vi "Info.vi"(8 "error in":errorcluster, 11 "VISA resource name":refnum<visa-resource-name>) -> (0 "error out\n(to Instr. Write/Read.vi)":errorcluster, 3 "VISA resource name out":refnum<visa-resource-name>)   [LabVIEW 2016, in "Agilent 415X Series.lvlib"]
doc: "This VI describes how to perform parameter range error checking if the user so desires to implement it."
uses:
  Agilent 415X Series.lvlib
panel:
  in  "x control":dbl format="%.2f"
  in  "revision history":string
  in  "by":string="Instrument Driver Development Team, National Instruments"
  in  "options":string="none (no HP16440A, HP16441A, HP16442A, or HP41501A"
  in  "comminication":u16(ring) items=["GPIB", "VXIbus", "Serial"]
  in  "firmware revision (*IDN?)":string="01.00:01.00:01.00"
  in  "manual revision or p/n":string="PN 04155-90120"
  in  "?":string="HP4155A Semiconductor Parameter Analyzer"
  # "instrument"
  # "instrument driver"
  # "more ..\n(see diagram)"
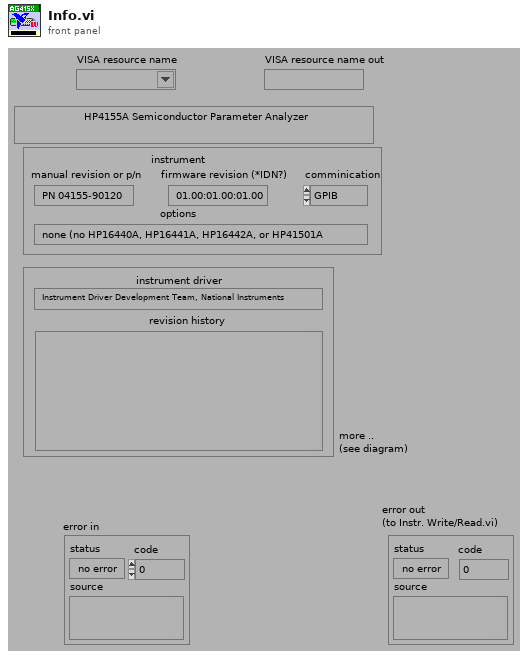
[diagram p1: front panel]
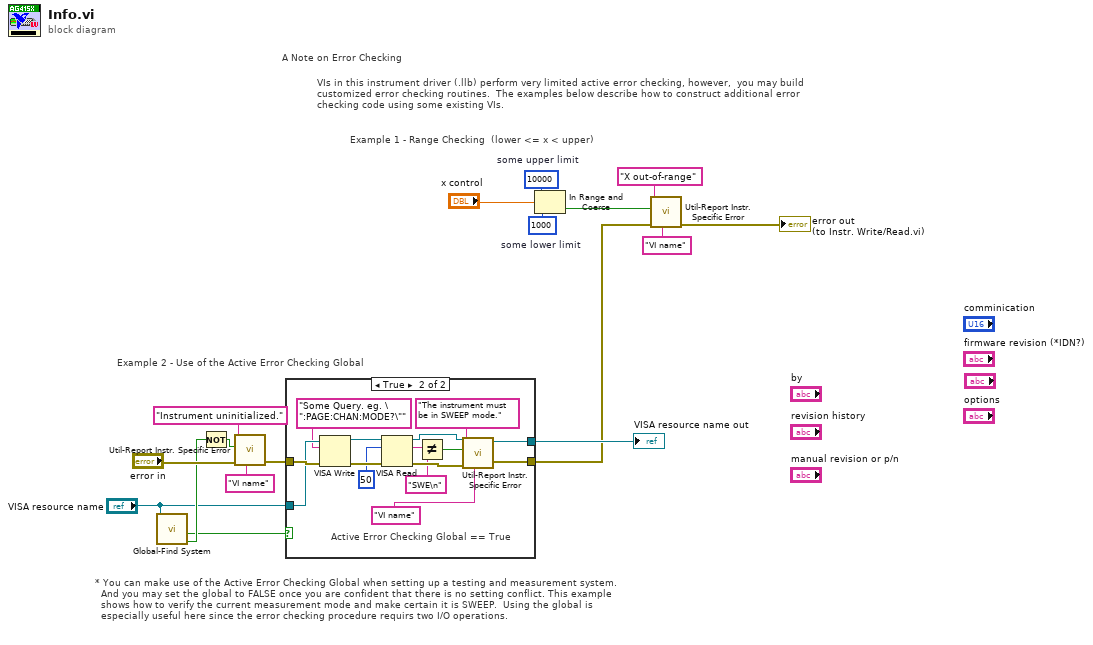
[diagram p0: block diagram]
diagram:
  w13 = 1000  # some lower limit
  w12 = 10000  # some upper limit
  # "A Note on Error Checking"
  # "* You can make use of the Active Error Checking Global when setting up a testing and measurement system.\n  And you may set the global to FALSE once you are confident that there is no setting conflict. This example\n  shows how to verify the current measurement mode and make certain it is SWEEP.  Using the global is  \n  especially useful here since the error checking procedure requirs two I/O operations."
  # "Example 2 - Use of the Active Error Checking Global"
  # "Example 1 - Range Checking  (lower <= x < upper)"
  # "VIs in this instrument driver (.llb) perform very limited active error checking, however,  you may build\ncustomized error checking routines.  The examples below describe how to construct additional error\nchecking code using some existing VIs."
  n1 = call "Global-Find System.vi"("VISA session"="VISA resource name") -> ("found"=w9:bool, "active error checking"=w6:bool)  [unwired: 3 in, 6 out]
  n2 = Not(x=w9) -> (.not. x?=w10:bool)
  n3 = call "Util-Report Instr. Specific Error.vi"("source"="VI name", "error in (no error)"="error in", "error message"="Instrument uninitialized.", "new error"=w10) -> ("error out"=w5:errorcluster)  [unwired: 6 in, 1 out]
  n4 = case shown="True" w6 {
    tunnel: w5 -> [w19 w34]
    tunnel: [w19 w25] -> w2
    tunnel: "VISA resource name" -> [w18 w32]
    tunnel: [w18 w20] -> w3
    frame False {
      # "Active Error Checking Global == False"
    }
    frame True {
      # "Active Error Checking Global == True"
      n5 = VISA Write(VISA resource name=w32, write buffer="Some Query. eg. \":PAGE:CHAN:MODE?\"", error in (no error)=w34) -> (VISA resource name out=w31:refnum<visa-resource-name>, error out=w33:errorcluster)  [unwired: 1 out]
      n6 = VISA Read(VISA resource name=w31, byte count=50, error in (no error)=w33) -> (VISA resource name out=w21:refnum<visa-resource-name>, read buffer=w28:string, error out=w26:errorcluster)  [unwired: 1 out]
      n7 = Not Equal?(x=w28, y="SWE\n") -> (x != y?=w27:bool)
      n8 = call "Util-Report Instr. Specific Error.vi"("source"="VI name", "error in (no error)"=w26, "error message"="The instrument must be in SWEEP mode.", "new error"=w27, "VISA resource name"=w21) -> ("error out"=w25:errorcluster, "VISA resource name out"=w20:refnum<visa-resource-name>)  [unwired: 5 in]
    }
  }
  "VISA resource name out" <- w3
  n9 = In Range and Coerce(upper limit=w12, x="x control", lower limit=w13) -> (In Range?=w17:bool)  [unwired: 1 out]
  n10 = call "Util-Report Instr. Specific Error.vi"("source"="VI name", "error in (no error)"=w2, "error message"="X out-of-range", "new error"=w17) -> ("error out"=→"error out\n(to Instr. Write/Read.vi)":errorcluster)  [unwired: 6 in, 1 out]
